vi "Open VI.vi"(7 "Open FP":bool, 11 "VI Path":path) -> (0 "error out":errorcluster, 3 "VI":refnum<vi>)   [LabVIEW 2020, in "NoCodeEngine.lvlib"]
uses:
  NoCodeEngine.lvlib
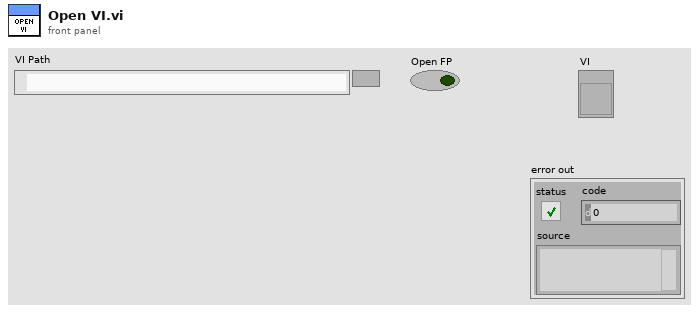
[diagram p1: front panel]
types:
  T1 = enum32{"Invalid", "Standard", "Closed", "Hidden", "Minimized", "Maximized"}
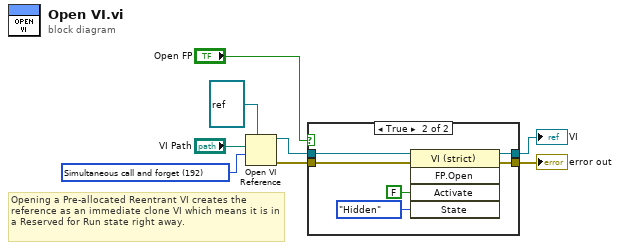
[diagram p0: block diagram]
diagram:
  w8 = 192 items=["Record modifications"=1, "Open templates for editing"=2, "Prompt user to save"=4, "Prepare for reentrant run"=8, "Prompt to find missing subVIs"=16, "Hide loading dialog box"=32, "Enable simultaneous calls"=64, "Prepare to call and forget"=128, "Simultaneous call and forget"=192, "Prepare to call and collect"=256, "Simultaneous call and collect"=320]
  # "Opening a Pre-allocated Reentrant VI creates the reference as an immediate clone VI which means it is in a Reserved for Run state right away."
  n1 = Open VI Reference(type specifier VI Refnum (for type only)=refnum<vi> refnum, vi path="VI Path", options=w8) -> (vi reference=w4:refnum<vi>, error out=w5:errorcluster)  [unwired: 3 in]
  n2 = case shown="True" "Open FP" {
    tunnel: w5 -> [w9 w16]
    tunnel: w4 -> [w10 w15]
    tunnel: [w10 w12] -> w1
    tunnel: [w9 w11] -> w2
    frame False {
    }
    frame True {
      n3 = invoke class="VI (strict)" method="FP.Open"(reference=w15, error in=w16, "Activate"=FALSE ("Activate?"), "State"=T1."Hidden") -> (reference out=w12:refnum<vi>, error out=w11:errorcluster)  [unwired: 1 in, 3 out]
    }
  }
  "error out" <- w2
  "VI" <- w1
